vi "Create Subscriber of Actor.vi"(8 "error in (no error)":errorcluster, 10 "Subscriber In":refnum<class "Subscriber.lvclass">, 11 "Mail Strategy in":refnum<class "Mail Strategy.lvclass">) -> (0 "error out":errorcluster, 2 "Subscriber Out":refnum<class "Subscriber.lvclass">, 3 "Mail Strategy out":refnum<class "Mail Strategy.lvclass">)   [LabVIEW 2024, in "Mail Strategy.lvclass"]
uses:
  Mail Strategy.lvclass
  Actor Assistant/Subscriber/Subscriber.lvclass
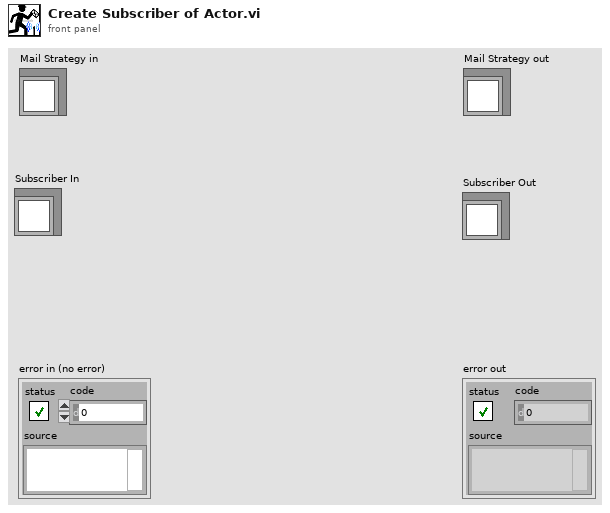
[diagram p1: front panel]
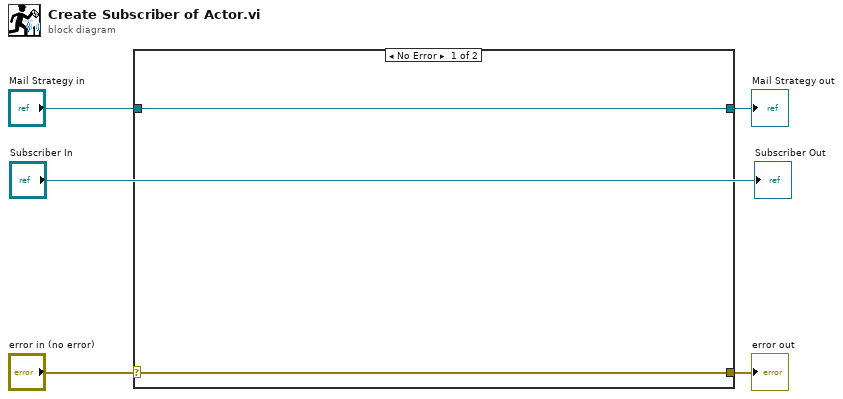
[diagram p0: block diagram]
diagram:
  n1 = case shown="No Error" "error in (no error)" {
    selector: "error in (no error)" -> [w6 w9]
    tunnel: [w6 w9] -> w4
    tunnel: [w7 w8] -> w2
    tunnel: "Mail Strategy in" -> [w7 w8]
    frame No Error {
    }
    frame Error {
    }
  }
  "error out" <- w4
  "Mail Strategy out" <- w2
  "Subscriber Out" <- "Subscriber In"
